vi "DrawBackground.vi"(8 "error in (no error)":errorcluster, 11 "Snake in":refnum<class "Snake.lvclass">) -> (0 "error out":errorcluster, 3 "Snake out":refnum<class "Snake.lvclass">)   [LabVIEW 2019, in "RT_Game.lvlib" / "Snake.lvclass"]
uses:
  Snake.lvclass
  C:/Users/FreshBob/Dropbox/VIs/myRIO_VGA/Classes/Game/Game.lvclass
  Snake.lvclass/Snake.ctl
  Game/Game.lvclass
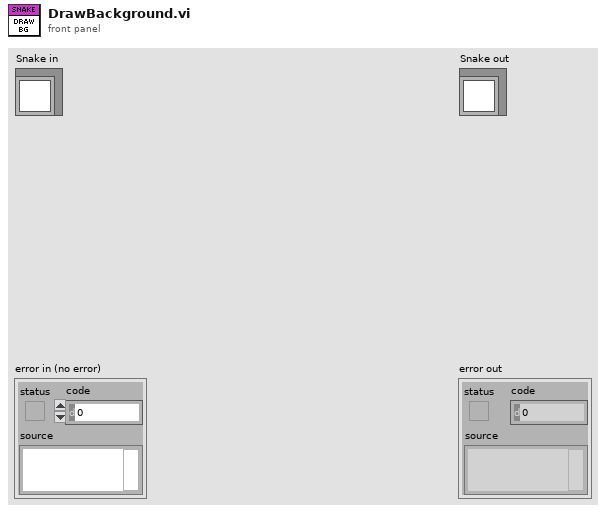
[diagram p1: front panel]
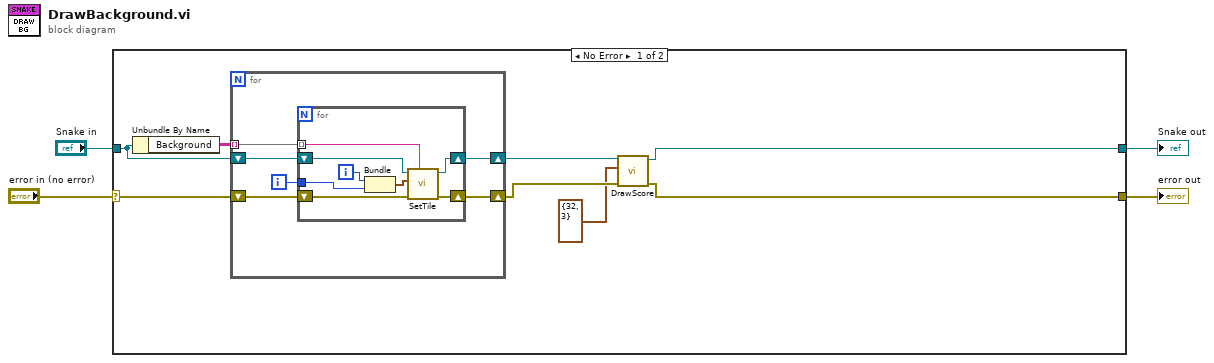
[diagram p0: block diagram]
diagram:
  n1 = case shown="No Error" "error in (no error)" {
    selector: "error in (no error)" -> [w10 w28]
    tunnel: [w8 w28] -> w3
    tunnel: [w5 w27] -> w1
    tunnel: "Snake in" -> [w11 w27]
    frame No Error {
      n2 = Unbundle By Name(w11) -> ("Background"=w12:string[][])
      n3 = for {
        tunnel: w12 -> [w18] mode=indexing
        shift-right: [w16] -> w7
        shift-left: w11 -> [w17]
        shift-right: [w15] -> w9
        shift-left: w10 -> [w14]
        i -> [w13]
        n4 = for {
          tunnel: w18 -> [w19] mode=indexing
          shift-right: [w25] -> w16
          shift-left: w17 -> [w26]
          shift-right: [w24] -> w15
          shift-left: w14 -> [w23]
          tunnel: w13 -> [w22]
          i -> [w21]
          n5 = Bundle(w21, w22) -> (w20:cluster{i32, i32})  [unwired: 1 in]
          n6 = call "SetTile.vi"("TileCode"=w19, "error in (no error)"=w23, "Coordinates"=w20, "Game in"=w26) -> ("error out"=w24:errorcluster, "Game out"=w25:refnum<class "Snake.lvclass">)  [unwired: 6 in]
        }
      }
      n7 = call "DrawScore.vi"("error in (no error)"=w9, "Coordinates"=cluster{"index_x":i32, "index_y":i32} {"index_x"=32, "index_y"=3}, "Snake in"=w7) -> ("error out"=w8:errorcluster, "Snake out"=w5:refnum<class "Snake.lvclass">)  [unwired: 7 in]
    }
    frame Error {
    }
  }
  "error out" <- w3
  "Snake out" <- w1
